vi "AB_RW_Project_DestinationItems.vi"(6 "usedDestinations":i32[](array[numeric]), 7 "action":T2, 8 "error in (no error)":errorcluster, 9 "buildTypeGUID":string, 10 "oldBuildObject":T1, 11 "buildObject":T1) -> (0 "error out":errorcluster, 3 "buildObject out":T1)   [LabVIEW 2020]
doc: "Reads and writes the data to the object property bag."
uses:
  <vilib>/AppBuilder/RW_Project/AB_RW_Project_PropBag_Action.ctl
  <vilib>/AppBuilder/RW_Project/AB_RW_Project_PropBag_ArrayAction.ctl
  <resource>/Framework/Providers/API/ItemRef.ctl
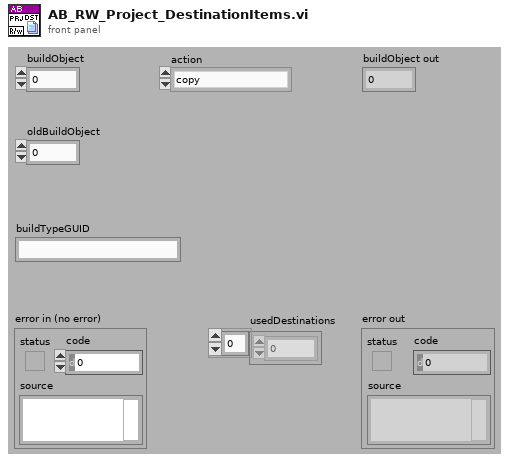
[diagram p1: front panel]
types:
  T1 = typedef "ItemRef.ctl" = u64
  T2 = typedef "AB_RW_Project_PropBag_ArrayAction.ctl" = enum16{"copy", "saveForPrevious", "loadFromPrevious", "clear"}
  T3 = typedef "AB_RW_Project_PropBag_Action.ctl" = enum16{"read", "write", "clear", "readPrevious", "writePrevious", "clearPrevious"}
  T4 = typedef "AB_RW_Project_Destination_Data.ctl" = cluster{"destName":string, "path":path, "preserveHierarchy":bool, "libraryName":string}
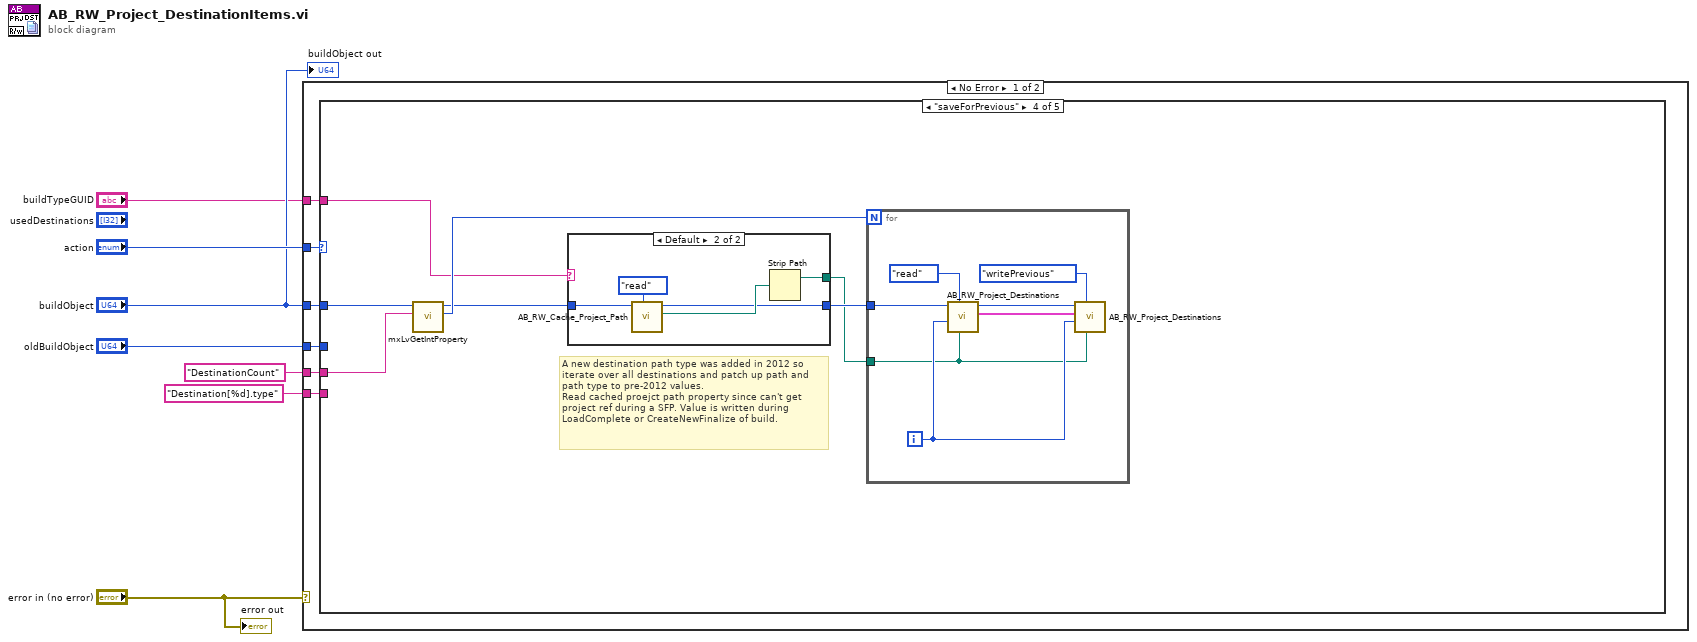
[diagram p0: block diagram]
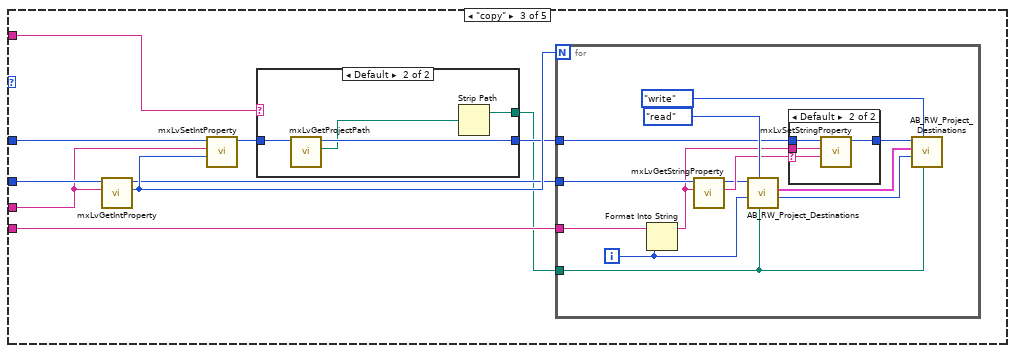
[diagram p4: hidden frame]
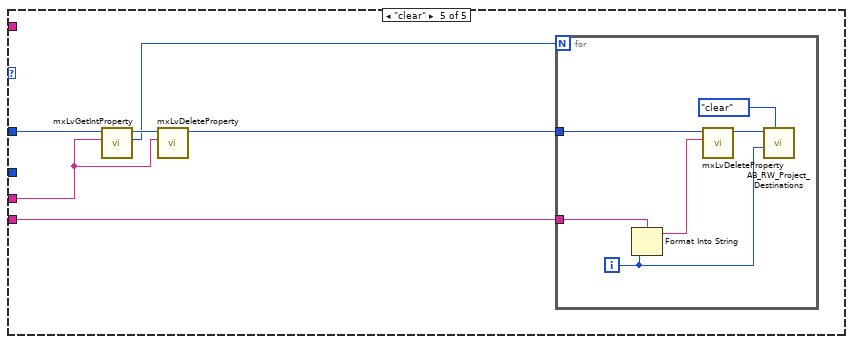
[diagram p8: hidden frame]
diagram:
  n1 = case shown="No Error" "error in (no error)" {
    tunnel: "action" -> [w13 _]
    tunnel: "buildObject" -> [w12 _]
    tunnel: "DestinationCount" -> [w11 _]
    tunnel: "Destination[%d].type" -> [w10 _]
    tunnel: "oldBuildObject" -> [w9 _]
    tunnel: "buildTypeGUID" -> [w8 _]
    frame No Error {
      n2 = case shown="\"saveForPrevious\"" w13 {
        tunnel: w12 -> [_ _ w19 w52 w72]
        tunnel: w11 -> [_ _ w20 w51 w69]
        tunnel: w10 -> [_ _ w23 _ w67]
        tunnel: w9 -> [_ _ w21 _ _]
        tunnel: w8 -> [_ _ w14 w48 _]
        frame Default {
        }
        frame "loadFromPrevious" {
        }
        frame "copy" {
          n3 = call <resource>:"mxLvGetIntProperty.vi"("Tag"=w20, "Item"=w21) -> ("Value"=w22:i32, "Item"=w18:T1)  [unwired: 7 in, 1 out]
          n4 = call <resource>:"mxLvSetIntProperty.vi"("Value (0)"=w22, "Tag"=w20, "Item"=w19) -> ("Item"=w17:T1)  [unwired: 7 in, 1 out]
          n5 = case shown="Default" w14 {
            tunnel: w17 -> [w24 w27]
            tunnel: [w24 w26] -> w16
            tunnel: [_ w28] -> w15
            frame "{69A947D5-514E-4E75-818E-69657C0547D8}" {
              # "For RTEXE, destination items are saved as absolute"
            }
            frame Default {
              n6 = call <resource>:"mxLvGetProjectPath.vi"("Item"=w27) -> ("Project Path"=w25:path, "Item"=w26:T1)  [unwired: 8 in, 1 out]
              n7 = Strip Path(path=w25) -> (stripped path=w28:path)  [unwired: 1 out]
            }
          }
          n8 = for {
            N: w22 -> [_]
            tunnel: w16 -> [w34]
            tunnel: w23 -> [w40]
            tunnel: w18 -> [w37]
            tunnel: w15 -> [w29]
            i -> [w30]
            n9 = Format Into String(format string=w40, w30) -> (resulting string=w36:string)  [unwired: 2 in, 1 out]
            n10 = call <resource>:"mxLvGetStringProperty.vi"("Tag"=w36, "Item"=w37) -> ("Value"=w35:string, "Item"=w33:T1)  [unwired: 7 in, 1 out]
            n11 = call <vilib>:"AB_RW_Project_Destinations.vi"("ProjectPath"=w29, "action"=AB_RW_Project_PropBag_Action."read", "index"=w30, "buildObject"=w33) -> ("index out"=w31:i32, "data out"=w32:T4)  [unwired: 4 in, 2 out]
            n12 = case shown="Default" w35 {
              selector: w35 -> [_ w43]
              tunnel: w34 -> [w42 w46]
              tunnel: w36 -> [_ w45]
              tunnel: [w42 w44] -> w39
              frame "" {
              }
              frame Default {
                n13 = call <resource>:"mxLvSetStringProperty.vi"("Value (\"\")"=w43, "Tag"=w45, "Item"=w46) -> ("Item"=w44:T1)  [unwired: 7 in, 1 out]
              }
            }
            n14 = call <vilib>:"AB_RW_Project_Destinations.vi"("ProjectPath"=w29, "action"=AB_RW_Project_PropBag_Action."write", "index"=w31, "data in"=w32, "buildObject"=w39) -> ()  [unwired: 3 in, 4 out]
          }
        }
        frame "saveForPrevious" {
          # "A new destination path type was added in 2012 so iterate over all destinations and patch up path and path type to pre-2012 values. \nRead cached proejct path property since can't get project ref during a SFP. Value is written during LoadComplete or CreateNewFinalize of build."
          n15 = call <resource>:"mxLvGetIntProperty.vi"("Tag"=w51, "Item"=w52) -> ("Value"=w53:i32, "Item"=w50:T1)  [unwired: 7 in, 1 out]
          n16 = case shown="Default" w48 {
            tunnel: w50 -> [w54 w56]
            tunnel: [w54 w55] -> w49
            tunnel: [_ w59] -> w47
            frame "{69A947D5-514E-4E75-818E-69657C0547D8}" {
              # "For RTEXE, destination items are saved as absolute"
            }
            frame Default {
              n17 = call <vilib>:"AB_RW_Cache_Project_Path.vi"("action"=AB_RW_Project_PropBag_Action."read", "buildObject"=w56) -> ("ProjectPath out"=w57:path, "buildObject out"=w55:T1)  [unwired: 7 in, 1 out]
              n18 = Strip Path(path=w57) -> (stripped path=w59:path)  [unwired: 1 out]
            }
          }
          n19 = for {
            N: w53 -> [_]
            tunnel: w49 -> [w65]
            tunnel: w47 -> [w61]
            i -> [w62]
            n20 = call <vilib>:"AB_RW_Project_Destinations.vi"("ProjectPath"=w61, "action"=AB_RW_Project_PropBag_Action."read", "index"=w62, "buildObject"=w65) -> ("data out"=w60:T4, "buildObject out"=w64:T1)  [unwired: 4 in, 2 out]
            n21 = call <vilib>:"AB_RW_Project_Destinations.vi"("ProjectPath"=w61, "action"=AB_RW_Project_PropBag_Action."writePrevious", "index"=w62, "data in"=w60, "buildObject"=w64) -> ()  [unwired: 3 in, 4 out]
          }
        }
        frame "clear" {
          n22 = call <resource>:"mxLvGetIntProperty.vi"("Tag"=w69, "Item"=w72) -> ("Value"=w70:i32, "Item"=w71:T1)  [unwired: 7 in, 1 out]
          n23 = call <resource>:"mxLvDeleteProperty.vi"("Tag"=w69, "Item"=w71) -> ("Item"=w68:T1)  [unwired: 8 in, 1 out]
          n24 = for {
            N: w70 -> [_]
            tunnel: w68 -> [w77]
            tunnel: w67 -> [w75]
            i -> [w74]
            n25 = Format Into String(format string=w75, w74) -> (resulting string=w73:string)  [unwired: 2 in, 1 out]
            n26 = call <resource>:"mxLvDeleteProperty.vi"("Tag"=w73, "Item"=w77) -> ("Item"=w76:T1)  [unwired: 8 in, 1 out]
            n27 = call <vilib>:"AB_RW_Project_Destinations.vi"("action"=AB_RW_Project_PropBag_Action."clear", "index"=w74, "buildObject"=w76) -> ()  [unwired: 5 in, 4 out]
          }
        }
      }
    }
    frame Error {
    }
  }
  "error out" <- "error in (no error)"
  "buildObject out" <- "buildObject"
